vi "Set Defaults.vi"(11 "NewEntityTemplate in":refnum<class "Test1.lvclass">) -> (3 "NewEntityTemplate out":refnum<class "Test1.lvclass">)   [LabVIEW 2020, in "tests.lvlib" / "Test1.lvclass"]
uses:
  Test1.lvclass
  Test1.lvclass/Test1.ctl
  <vilib>/IlluminatedG/IG Conditum Base/Conditum/Columns/Integer/Integer.lvclass
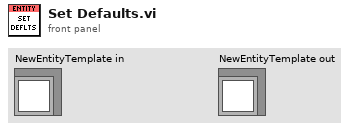
[diagram p1: front panel]
types:
  T1 = typedef "tests.lvlib/Test1.lvclass/Columns.ctl" = cluster{"<Placeholder>":refnum<class "Integer.lvclass">}
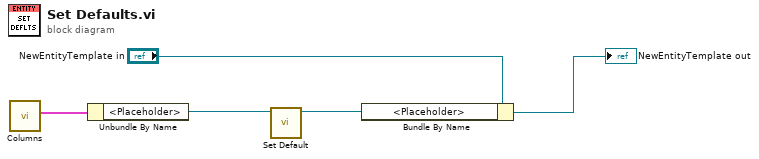
[diagram p0: block diagram]
diagram:
  n1 = call "Columns.vi"() -> ("Columns"=w5:T1)  [unwired: 11 in]
  n2 = Unbundle By Name(w5) -> ("<Placeholder>"=w4:refnum<class "Integer.lvclass">)
  n3 = call-dynamic "Set Default.vi"("Integer in"=w4) -> ("Integer out"=w2:refnum<class "Integer.lvclass">)  [unwired: 10 in]
  n4 = Bundle By Name(cluster="NewEntityTemplate in", "<Placeholder>"=w2) -> (→"NewEntityTemplate out":refnum<class "Test1.lvclass">)
